vi "FTW-Container-Object-Insert.vi"(0 "Object in":T1, 5 "Element Name":string, 7 "Container":variant) -> (4 "?":T1, 10 "Found":bool)   [LabVIEW 2015, in "FTW-Container.lvclass"]
uses:
  FTW-Container.lvclass
  FTW-Container-Object.ctl
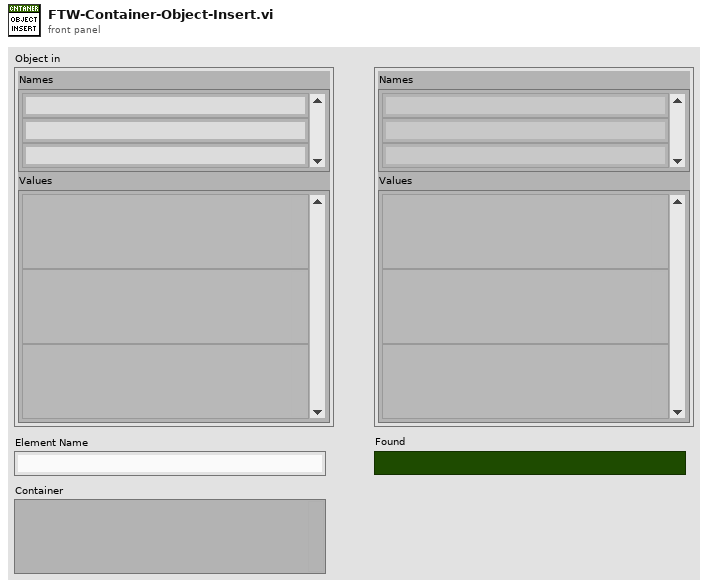
[diagram p1: front panel]
types:
  T1 = typedef "FTW-Container.lvclass/FTW-Container-Object.ctl" = cluster{"Names":string[], "Values":variant[]}
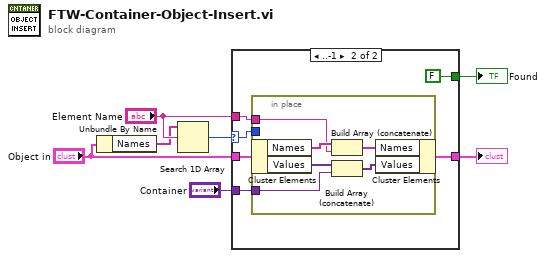
[diagram p0: block diagram]
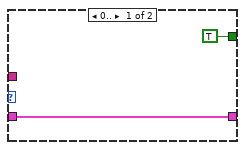
[diagram p2: hidden frame]
diagram:
  n1 = Unbundle By Name("Object in") -> ("Names"=w1:string[])
  n2 = Search 1D Array(1D array=w1, element="Element Name") -> (index of element=w2:i32)  [unwired: 1 in]
  n3 = case shown="..-1" w2 {
    selector: w2 -> [_ w11]
    tunnel: "Container" -> [_ w15]
    tunnel: "Element Name" -> [_ w14]
    tunnel: [w9 w13] -> w5
    tunnel: "Object in" -> [w9 w12]
    tunnel: [TRUE FALSE] -> w3
    frame 0.. {
    }
    frame ..-1 {
      n4 = in-place {
        in-place-border: w11 -> [_]
        in-place-border: w14 -> [w17]
        in-place-border: w15 -> [w16]
        n5 = in-place-cluster #1(w12) -> ("Names"=w21:string[], "Values"=w19:variant[])
        n6 = Build Array (concatenate)(w21, w17) -> (w20:string[])
        n7 = Build Array (concatenate)(w19, w16) -> (w18:variant[])
        n8 = in-place-cluster #1("Names"=w20, "Values"=w18) -> (w13:T1)
      }
    }
  }
  "?" <- w5
  "Found" <- w3
